vi "Event Handler.vi"(8 "error in (no error)":errorcluster, 10 "Stop Event Handler":refnum<user-event>, 11 "SingleStepTestV3 in":refnum<class "SingleStepCODMnV2.lvclass">) -> (0 "error out":errorcluster)   [LabVIEW 2016, in "SingleStepCODMnV2.lvlib" / "SingleStepCODMnV2.lvclass"]
doc: "The <b>Event Handler VI</b> is a dynamic dispatch VI that should be overwritten if events are needed to create the enhanced QControl. \n\nBy inheriting from the main Control.lvclass the overwritten <b>Event Handler VI</b> will be launched asynchronously in the initialization of the QControl.\n<b> </b> <b> </b>\n©2016 Q Software Innovations, LLC (QSI)\nwritten by Quentin Alldredge\nproduced in LabVIEW 2015\n\nsupport@qsoftwareinnovations.com\nwww.qsoftwareinnovations.com\n\nAll rights reserved.\n\nRedistribution and use in source and binary forms, with or without modification, are permitted provided that the following conditions are met:\n\n * Redistributions of source code must retain the above copyright notice, this list of conditions and the following disclaimer.\n * Redistributions in binary form must reproduce the above copyright notice, this list of conditions and the following disclaimer in the documentation and/or other materials provided with the distribution.\n * Neither the name of Q Software Innovations, LLC. nor the names of its contributors may be used to endorse or promote products derived from this software without specific prior written permission.\n\nTHIS SOFTWARE IS PROVIDED BY THE COPYRIGHT HOLDERS AND CONTRIBUTORS \"AS IS\" AND ANY EXPRESS OR IMPLIED WARRANTIES, INCLUDING, BUT NOT LIMITED TO, THE IMPLIED WARRANTIES OF MERCHANTABILITY AND FITNESS FOR A PARTICULAR PURPOSE ARE DISCLAIMED. IN NO EVENT SHALL THE COPYRIGHT OWNER OR CONTRIBUTORS BE LIABLE FOR ANY DIRECT, INDIRECT, INCIDENTAL, SPECIAL, EXEMPLARY, OR CONSEQUENTIAL DAMAGES (INCLUDING, BUT NOT LIMITED TO, PROCUREMENT OF SUBSTITUTE GOODS OR SERVICES; LOSS OF USE, DATA, OR PROFITS; OR BUSINESS INTERRUPTION) HOWEVER CAUSED AND ON ANY THEORY OF LIABILITY, WHETHER IN CONTRACT, STRICT LIABILITY, OR TORT (INCLUDING NEGLIGENCE OR OTHERWISE) ARISING IN ANY WAY OUT OF THE USE OF THIS SOFTWARE, EVEN IF ADVISED OF THE POSSIBILITY OF SUCH DAMAGE."
uses:
  SingleStepCODMnV2.lvclass
  SingleStepCODMnV2.lvclass/SingleStepCODMnV2.ctl
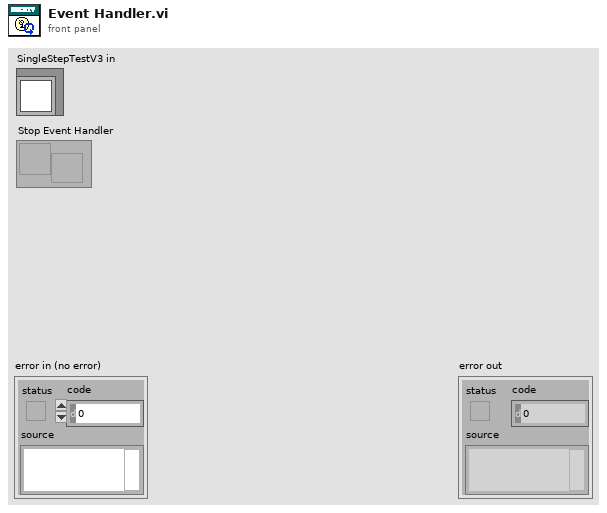
[diagram p1: front panel]
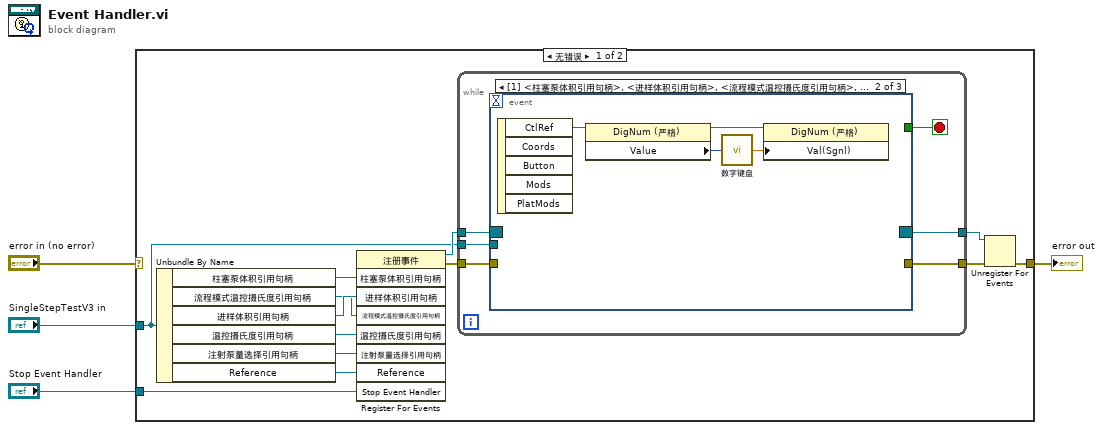
[diagram p0: block diagram]
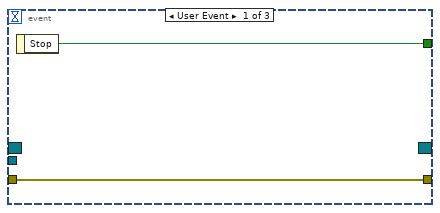
[diagram p2: hidden frame]
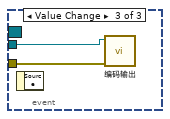
[diagram p3: hidden frame]
diagram:
  n1 = case shown="无错误" "error in (no error)" {
    selector: "error in (no error)" -> [_ w32]
    tunnel: [w14 w32] -> w3
    tunnel: "SingleStepTestV3 in" -> [w12 _]
    tunnel: "Stop Event Handler" -> [w11 _]
    frame No Error {
      n2 = Unbundle By Name(w12) -> ("柱塞泵体积引用句柄"=w10:refnum<vi>, "流程模式温控摄氏度引用句柄"=w5:refnum<vi>, "进样体积引用句柄"=w9:refnum<vi>, "温控摄氏度引用句柄"=w8:refnum<vi>, "注射泵量选择引用句柄"=w7:refnum<vi>, "Reference"=w6:refnum<vi>)
      n3 = register-events(w10, w9, w5, w8, w7, w6, w11) -> (reference out=w17:refnum<event-registration>, error out=w16:errorcluster)  [unwired: 2 in]
      n4 = while {
        tunnel: w17 -> [w23]
        tunnel: w16 -> [w21]
        tunnel: [w20] -> w15
        tunnel: [w18] -> w13
        tunnel: w12 -> [w22]
        stop <- w19 stop-if-true
        n5 = event shown="[1] <柱塞泵体积引用句柄>, <进样体积引用句柄>, <流程模式温控摄氏度引用句柄>, <温控摄氏度引用句柄>, <注射泵量选择引用句柄>: 鼠标按下" {
          selector: w23 -> [_ _ _]
          dyn-events: [_ _ _] -> w18
          timeout: _ -> [_ _ _]
          tunnel: w22 -> [_ _ w31]
          tunnel: w21 -> [w25 _ w30]
          tunnel: [w25 _ _] -> w20
          tunnel: [w24 _ _] -> w19
          event User Event {
            n6 = event-data() -> ("Stop"=w24:bool)  [unwired: 1 in]
          }
          event Mouse Down {
            n7 = event-data() -> ("CtlRef"=w29:refnum<vi>)  [unwired: 1 in, 4 out]
            n8 = property class="DigNum (严格)"(reference=w29) -> (reference out=w27:refnum<vi>, "Value"=w28:u16)  [unwired: 1 in, 1 out]
            n9 = call "数字键盘.vi"("OldNumber"=w28) -> ("NewNumber"=w26:sgl)
            n10 = property class="DigNum (严格)"(reference=w27, "Val(Sgnl)"=w26) -> ()  [unwired: 1 in, 2 out]
          }
          event Value Change {
            n11 = event-data() -> ()  [unwired: 1 in, 1 out]
            n12 = call "编码输出.vi"("error in (no error)"=w30, "SingleStepTestV3输入"=w31) -> ()  [unwired: 8 in, 2 out]
          }
        }
      }
      n13 = Unregister For Events(event registration refnum=w13, error in=w15) -> (error out=w14:errorcluster)
    }
    frame Error {
    }
  }
  "error out" <- w3
